vi "Create Server.vi"(8 "error in (no error)":errorcluster) -> (0 "error out":errorcluster, 3 "Server":refnum<class "Server.lvclass">)   [LabVIEW 2020, in "Server.lvlib"]
doc: "Create a PVAccess server."
uses:
  Server.lvlib
  Server/Server.lvclass
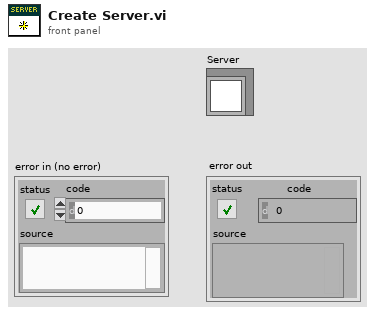
[diagram p1: front panel]
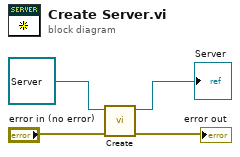
[diagram p0: block diagram]
diagram:
  n1 = call "Create.vi"("error in (no error)"="error in (no error)", "Server in"=refnum<class "Server.lvclass"> refnum ("Server.lvlib:Server.lvclass")) -> ("error out"=→"error out":errorcluster, "Server out"=→"Server":refnum<class "Server.lvclass">)  [unwired: 8 in]
